vi "Get Times.vi"() -> (0 "Array [time {ms}, distance, anchor id]":string[][](array[string]))   [LabVIEW 2014, in "Position.lvclass"]
uses:
  Position.lvclass
panel:
  out "Input":string[][](array[string])
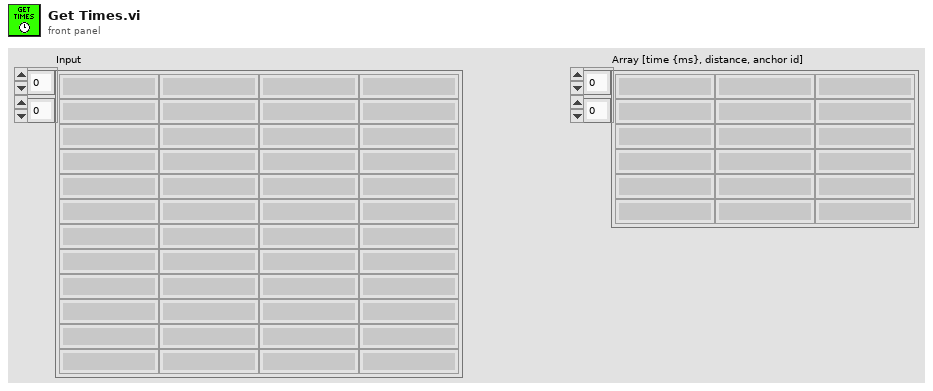
[diagram p1: front panel]
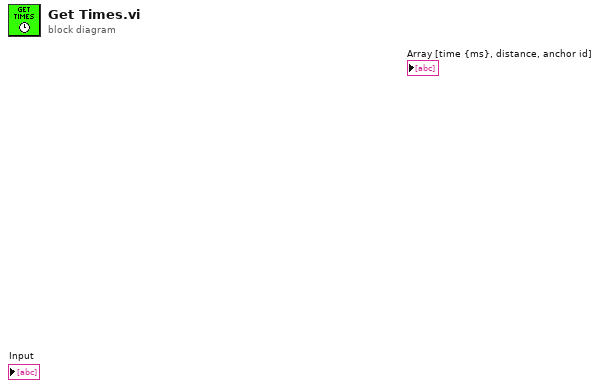
[diagram p0: block diagram]
diagram:
